vi "WriteData.vi"(8 "Error In":errorcluster, 10 "Data":string, 11 "reference in":refnum<class "EncryptionDecorator.lvclass">) -> (0 "Error Out":errorcluster, 3 "reference in":refnum<class "EncryptionDecorator.lvclass">)   [LabVIEW 2020, in "EncryptionDecorator.lvclass"]
uses:
  EncryptionDecorator.lvclass
  DataSourceDecorator_class/DataSourceDecorator.lvclass
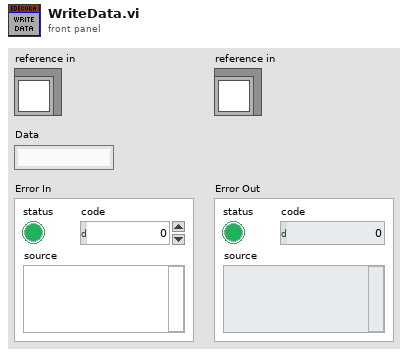
[diagram p1: front panel]
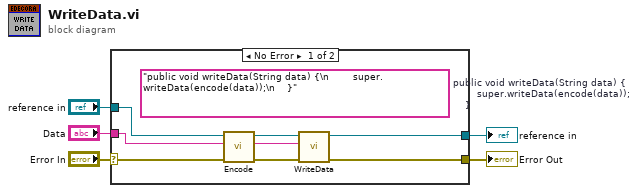
[diagram p0: block diagram]
diagram:
  n1 = case shown="No Error" "Error In" {
    selector: "Error In" -> [w8 w15]
    tunnel: [w12 w15] -> w4
    tunnel: [w13 w14] -> w2
    tunnel: "reference in" -> [w9 w14]
    tunnel: "Data" -> [w11 _]
    frame No Error {
      (unwired) "public void writeData(String data) {\n        super.writeData(encode(data));\n    }"  # public void writeData(String data) {         super.writeData(encode(data));     }
      n2 = call "Encode.vi"("Error In"=w8, "Data"=w11, "reference in"=w9) -> ("Error Out"=w7:errorcluster, "Return(STRING)"=w6:string, "reference in"=w10:refnum<class "EncryptionDecorator.lvclass">)  [unwired: 6 in]
      n3 = call-parent "WriteData.vi"("Error In"=w7, "Data"=w6, "reference in"=w10) -> ("Error Out"=w12:errorcluster, "reference out"=w13:refnum<class "EncryptionDecorator.lvclass">)  [unwired: 7 in]
    }
    frame Error {
    }
  }
  "Error Out" <- w4
  "reference in" <- w2
